vi "pH V to V20.vi"(1 "Temperature":dbl format="%.2f", 2 "Voltage":dbl format="%.2f") -> (0 "V20":dbl format="%.2f")   [LabVIEW 2010]
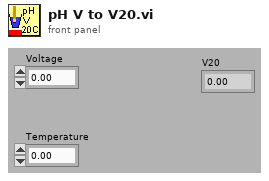
[diagram p1: front panel]
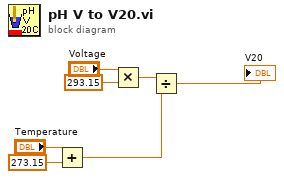
[diagram p0: block diagram]
diagram:
  n1 = Add(x="Temperature", y=273.15) -> (x+y=w2:dbl)
  n2 = Multiply(x="Voltage", y=293.15) -> (x*y=w3:dbl)
  n3 = Divide(x=w3, y=w2) -> (x/y=→"V20":dbl)
